vi "Linker.Find Tests and Suites.vi"(11 "Linker:Read Info From File":T2(array[cluster])) -> (1 "All VIs defining a Test Runner":path[](array[path]), 2 "All VIs defining a suite":path[](array[path]), 3 "All VIs defining a test (excluding those defining a suite)":path[](array[path]))   [LabVIEW 2013]
uses:
  <vilib>/Utility/lvfile.llb/LVFileType.ctl
  <vilib>/Utility/lvfile.llb/NI_FileType.lvlib
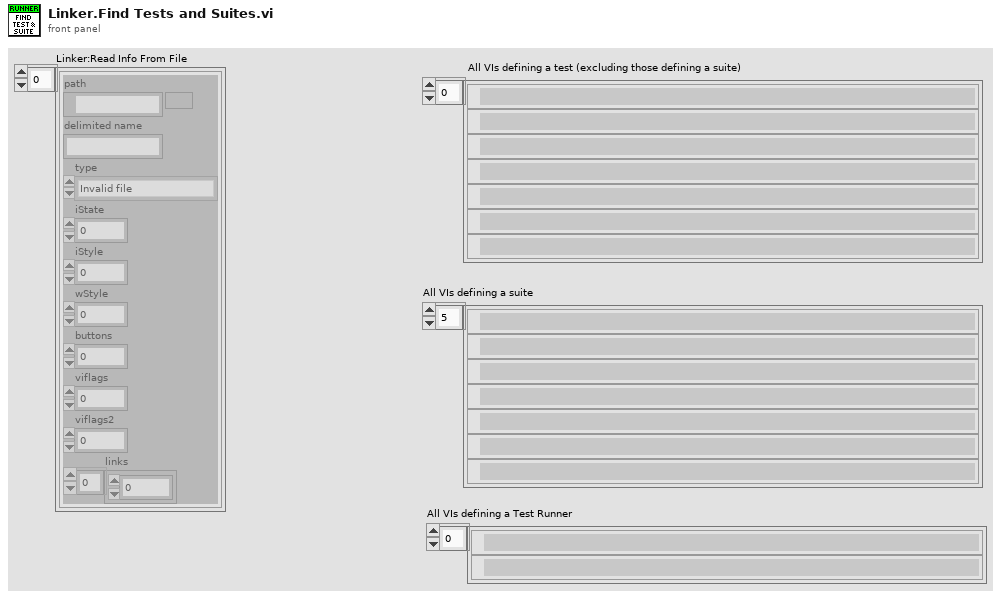
[diagram p1: front panel]
types:
  T1 = typedef "NI_FileType.lvlib/LVFileType.ctl" = enum32{"Invalid file", "Unknown type", "Instrument", "Control", "Polymorphic VI", "Project", "Library", "LVClass", "XControl", "XNode", "Shared library", ".NET assembly", "ActiveX interface", "CIN", "Run-time menu", "Palette menu", "Help file", "LLB", "XNode Edit Dependency", "Class Private Data Control", "Statechart", "MathScript .m file", "Ladder Diagram", "LVLibp", "XNode Build Dependency"}
  T2 = cluster{"path":path, "delimited name":string, "type":T1, "iState":u32, "iStyle":u16, "wStyle":u16, "buttons":u16, "viflags":u32, "viflags2":u32, "links":u32[]}[]
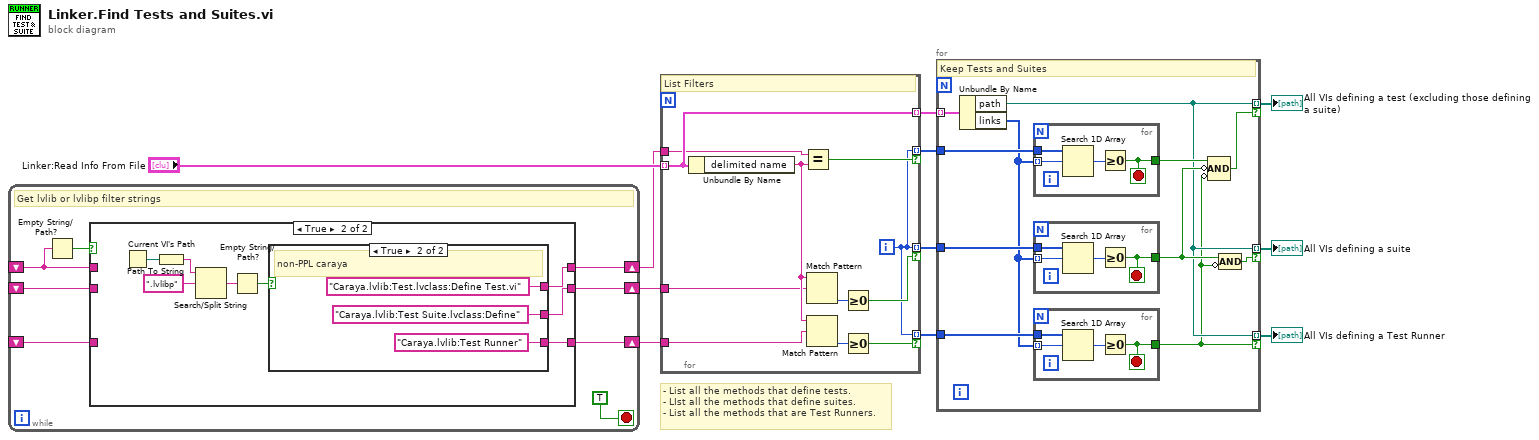
[diagram p0: block diagram]
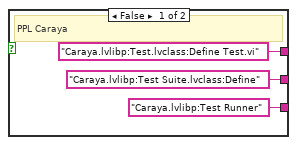
[diagram p3: hidden frame]
diagram:
  # "- List all the methods that define tests.\n- LIst all the methods that define suites.\n- List all the methods that are Test Runners."
  n1 = while {
    shift-right: [w19] -> w3
    shift-left: _ -> [w14]
    shift-right: [w18] -> w2
    shift-left: _ -> [w13]
    shift-right: [w17] -> w1
    shift-left: _ -> [w12]
    stop <- TRUE stop-if-true
    # "Get lvlib or lvlibp filter strings"
    n2 = Empty String/Path?(string/path=w14) -> (empty?=w15:bool)
    n3 = case shown="True" w15 {
      tunnel: [w22 w25] -> w19
      tunnel: [w21 w24] -> w18
      tunnel: [w20 w23] -> w17
      tunnel: w14 -> [w22 _]
      tunnel: w13 -> [w21 _]
      tunnel: w12 -> [w20 _]
      frame False {
      }
      frame True {
        n4 = Current VI's Path() -> (path=w30:path)
        n5 = Path To String(path=w30) -> (string=w29:string)
        n6 = Search/Split String(string=w29, search string/char (-)=".lvlibp") -> (match + rest of string=w27:string)  [unwired: 1 in, 2 out]
        n7 = Empty String/Path?(string/path=w27) -> (empty?=w26:bool)
        n8 = case shown="True" w26 {
          tunnel: ["Caraya.lvlibp:Test.lvclass:Define Test.vi" ("pattern") "Caraya.lvlib:Test.lvclass:Define Test.vi" ("pattern")] -> w25
          tunnel: ["Caraya.lvlibp:Test Suite.lvclass:Define" ("pattern") "Caraya.lvlib:Test Suite.lvclass:Define" ("pattern")] -> w24
          tunnel: ["Caraya.lvlibp:Test Runner" ("pattern") "Caraya.lvlib:Test Runner" ("pattern")] -> w23
          frame False {
            # "PPL Caraya"
          }
          frame True {
            # "non-PPL caraya"
          }
        }
      }
    }
  }
  n9 = for {
    tunnel: "Linker:Read Info From File" -> [w44] mode=indexing
    tunnel: [w42] -> w11 mode=indexing if=w46
    tunnel: [w42] -> w10 mode=indexing if=w45
    tunnel: [w44] -> w9 mode=indexing
    tunnel: [w42] -> w5 mode=indexing if=w41
    tunnel: w3 -> [w39]
    tunnel: w2 -> [w38]
    tunnel: w1 -> [w37]
    i -> [w42]
    # "List Filters"
    n10 = Unbundle By Name(w44) -> ("delimited name"=w40:string)
    n11 = Equal?(x=w39, y=w40) -> (x = y?=w46:bool)
    n12 = Match Pattern(string=w40, regular expression=w38) -> (offset past match=w47:i32)  [unwired: 1 in, 3 out]
    n13 = Match Pattern(string=w40, regular expression=w37) -> (offset past match=w43:i32)  [unwired: 1 in, 3 out]
    n14 = Greater Or Equal To 0?(x=w47) -> (x >= 0?=w45:bool)
    n15 = Greater Or Equal To 0?(x=w43) -> (x >= 0?=w41:bool)
  }
  n16 = for {
    tunnel: w9 -> [w54] mode=indexing
    tunnel: w11 -> [w58]
    tunnel: [w49] -> w7 mode=indexing if=w55
    tunnel: w10 -> [w57]
    tunnel: [w49] -> w6 mode=indexing if=w51
    tunnel: w5 -> [w53]
    tunnel: [w49] -> w4 mode=indexing if=w48
    # "Keep Tests and Suites"
    n17 = Unbundle By Name(w54) -> ("path"=w49:path, "links"=w52:u32[])
    n18 = for {
      tunnel: w58 -> [w70]
      tunnel: w52 -> [w69] mode=indexing
      tunnel: [w67] -> w56
      stop <- w67 stop-if-true
      n19 = Search 1D Array(1D array=w70, element=w69) -> (index of element=w68:i32)  [unwired: 1 in]
      n20 = Greater Or Equal To 0?(x=w68) -> (x >= 0?=w67:bool)
    }
    n21 = for {
      tunnel: w57 -> [w66]
      tunnel: w52 -> [w65] mode=indexing
      tunnel: [w63] -> w50
      stop <- w63 stop-if-true
      n22 = Search 1D Array(1D array=w66, element=w65) -> (index of element=w64:i32)  [unwired: 1 in]
      n23 = Greater Or Equal To 0?(x=w64) -> (x >= 0?=w63:bool)
    }
    n24 = for {
      tunnel: w53 -> [w62]
      tunnel: w52 -> [w61] mode=indexing
      tunnel: [w59] -> w48
      stop <- w59 stop-if-true
      n25 = Search 1D Array(1D array=w62, element=w61) -> (index of element=w60:i32)  [unwired: 1 in]
      n26 = Greater Or Equal To 0?(x=w60) -> (x >= 0?=w59:bool)
    }
    n27 = Compound Arithmetic op=AND(w56, invert w50, invert w48) -> (w55:bool)
    n28 = Compound Arithmetic op=AND(w50, invert w48) -> (w51:bool)
  }
  "All VIs defining a test (excluding those defining a suite)" <- w7
  "All VIs defining a suite" <- w6
  "All VIs defining a Test Runner" <- w4
